vi "Convert Array from BMIH.vi"(1 "BITMAPINFOHEADER":T1) -> (0 "Array":u8[](array[numeric]))   [LabVIEW 2013, in "VRI.lvlib"]
uses:
  VRI.lvlib
  _Type Defs/BITMAPINFOHEADER.ctl
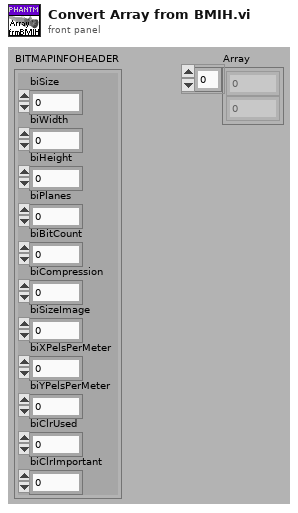
[diagram p1: front panel]
types:
  T1 = typedef "VRI.lvlib/BITMAPINFOHEADER.ctl" = cluster{"biSize":u32, "biWidth":i32, "biHeight":i32, "biPlanes":u16, "biBitCount":u16, "biCompression":u32, "biSizeImage":u32, "biXPelsPerMeter":i32, "biYPelsPerMeter":i32, "biClrUsed":u32, "biClrImportant":u32}
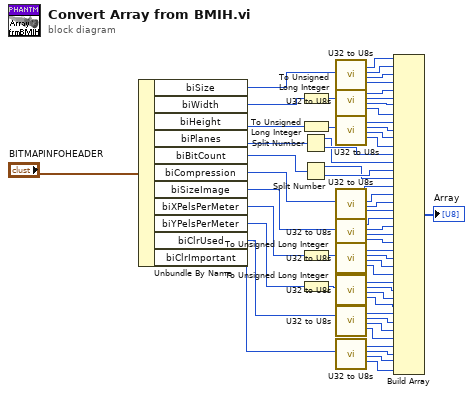
[diagram p0: block diagram]
diagram:
  n1 = Unbundle By Name("BITMAPINFOHEADER") -> ("biSize"=w2:u32, "biWidth"=w7:i32, "biHeight"=w14:i32, "biPlanes"=w19:u16, "biBitCount"=w22:u16, "biCompression"=w27:u32, "biSizeImage"=w36:u32, "biXPelsPerMeter"=w45:i32, "biYPelsPerMeter"=w46:i32, "biClrUsed"=w47:u32, "biClrImportant"=w48:u32)
  n2 = To Unsigned Long Integer(number=w7) -> (unsigned 32bit integer=w13:u32)
  n3 = To Unsigned Long Integer(number=w14) -> (unsigned 32bit integer=w12:u32)
  n4 = Split Number(x=w19) -> (hi(x)=w20:u8, lo(x)=w21:u8)
  n5 = Split Number(x=w22) -> (hi(x)=w23:u8, lo(x)=w24:u8)
  n6 = To Unsigned Long Integer(number=w45) -> (unsigned 32bit integer=w25:u32)
  n7 = To Unsigned Long Integer(number=w46) -> (unsigned 32bit integer=w26:u32)
  n8 = call "U32 to U8s.vi"("U32"=w2) -> ("HiHi"=w3:u8, "Hi"=w4:u8, "Lo"=w5:u8, "LoLo"=w6:u8)  [unwired: 15 out]
  n9 = call "U32 to U8s.vi"("U32"=w13) -> ("HiHi"=w8:u8, "Hi"=w9:u8, "Lo"=w10:u8, "LoLo"=w11:u8)  [unwired: 15 out]
  n10 = call "U32 to U8s.vi"("U32"=w12) -> ("HiHi"=w15:u8, "Hi"=w16:u8, "Lo"=w17:u8, "LoLo"=w18:u8)  [unwired: 15 out]
  n11 = call "U32 to U8s.vi"("U32"=w27) -> ("HiHi"=w28:u8, "Hi"=w29:u8, "Lo"=w30:u8, "LoLo"=w31:u8)  [unwired: 15 out]
  n12 = call "U32 to U8s.vi"("U32"=w36) -> ("HiHi"=w32:u8, "Hi"=w33:u8, "Lo"=w34:u8, "LoLo"=w35:u8)  [unwired: 15 out]
  n13 = call "U32 to U8s.vi"("U32"=w25) -> ("HiHi"=w37:u8, "Hi"=w38:u8, "Lo"=w39:u8, "LoLo"=w40:u8)  [unwired: 15 out]
  n14 = call "U32 to U8s.vi"("U32"=w26) -> ("HiHi"=w41:u8, "Hi"=w42:u8, "Lo"=w43:u8, "LoLo"=w44:u8)  [unwired: 15 out]
  n15 = call "U32 to U8s.vi"("U32"=w47) -> ("HiHi"=w49:u8, "Hi"=w50:u8, "Lo"=w51:u8, "LoLo"=w52:u8)  [unwired: 15 out]
  n16 = call "U32 to U8s.vi"("U32"=w48) -> ("HiHi"=w53:u8, "Hi"=w54:u8, "Lo"=w55:u8, "LoLo"=w56:u8)  [unwired: 15 out]
  n17 = Build Array(w3, w4, w5, w6, w8, w9, w10, w11, w15, w16, w17, w18, w21, w20, w24, w23, w28, w29, w30, w31, w32, w33, w34, w35, w37, w38, w39, w40, w41, w42, w43, w44, w49, w50, w51, w52, w53, w54, w55, w56) -> (→"Array":u8[])
